vi "Check Channel Pair (SubVI).vi"(6 "seconds to wait":u32=100, 7 "OutputChannel Value in":dbl, 8 "error in (no error)":errorcluster, 9 "Input Channel":string, 10 "Output Channel":string, 11 "WorkspaceManager in":T1) -> (0 "error out":errorcluster, 1 "OutputChannel Value out":dbl, 2 "InputChanel Value":dbl, 3 "WorkspaceManager out":T1)   [LabVIEW 2020, in "FPGA Addon Test Class.lvclass"]
uses:
  FPGA Addon Test Class.lvclass
  <vilib>/NI VeriStand/Execution/Workspace/WorkspaceAPI.ctl
  NationalInstruments.VeriStand.ClientAPI
  <vilib>/NI VeriStand/Execution/Workspace/NI VeriStand - Set Single Channel Value.vi
  <vilib>/NI VeriStand/Execution/Workspace/NI VeriStand - Get Single Channel Value.vi
  <vilib>/NI VeriStand/Execution/Workspace/NI_VS Workspace ExecutionAPI.lvlib
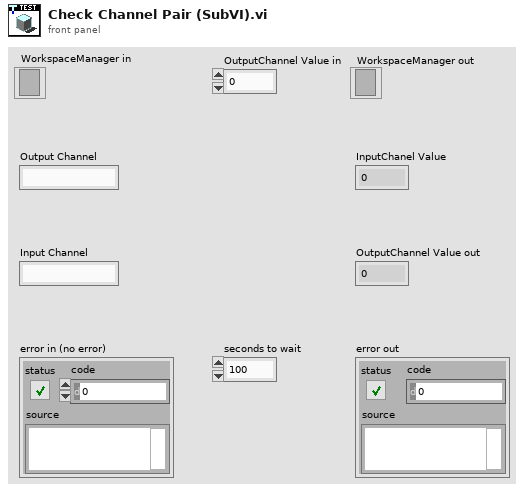
[diagram p1: front panel]
types:
  T1 = typedef "NI_VS Workspace ExecutionAPI.lvlib/WorkspaceAPI.ctl" = refnum<k24>
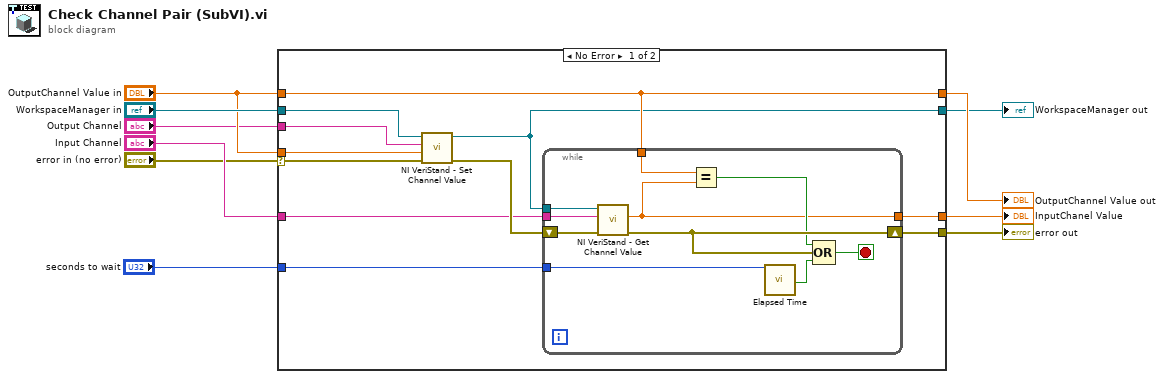
[diagram p0: block diagram]
diagram:
  n1 = case shown="No Error" "error in (no error)" {
    selector: "error in (no error)" -> [w16 w34]
    tunnel: "OutputChannel Value in" -> [w13 w33]
    tunnel: [w21 w34] -> w5
    tunnel: "Input Channel" -> [w19 _]
    tunnel: "OutputChannel Value in" -> [w18 _]
    tunnel: "WorkspaceManager in" -> [w17 w32]
    tunnel: "Output Channel" -> [w15 _]
    tunnel: "seconds to wait" -> [w14 _]
    tunnel: [w13 w33] -> w3
    tunnel: [w12 _] -> w2
    tunnel: [w11 w32] -> w1
    frame No Error {
      n2 = call-poly <vilib>:"NI VeriStand - Set Channel Value.vi"("error in (no error)"=w16, "Value"=w18, "Channel"=w15, "WorkspaceManager in"=w17) -> ("error out"=w20:errorcluster, "WorkspaceManager out"=w11:T1)  [unwired: 6 in]
      n3 = while {
        tunnel: w13 -> [w31]
        tunnel: w19 -> [w29]
        tunnel: w11 -> [w28]
        shift-right: [w26] -> w21
        shift-left: w20 -> [w30]
        tunnel: w14 -> [w23]
        tunnel: [w22] -> w12
        stop <- w25 stop-if-true
        n4 = call-poly <vilib>:"NI VeriStand - Get Channel Value.vi"("error in (no error)"=w30, "Channel"=w29, "WorkspaceManager in"=w28) -> ("error out"=w26:errorcluster, "Value"=w22:dbl)  [unwired: 6 in, 1 out]
        n5 = Equal?(x=w31, y=w22) -> (x = y?=w24:bool)
        n6 = call "Elapsed Time"("Time Target (s)"=w23) -> ("Time has Elapsed"=w27:bool)  [unwired: 11 in, 7 out]
        n7 = Compound Arithmetic op=OR(w24, w26, w27) -> (w25:bool)
      }
    }
    frame Error {
    }
  }
  "error out" <- w5
  "InputChanel Value" <- w2
  "OutputChannel Value out" <- w3
  "WorkspaceManager out" <- w1
